vi "Notifer ControlThread.vi"() -> ()   [LabVIEW 2015]
panel:
  out "Waveform Chart 2":dbl(graph)
  out "Waveform Chart":dbl(graph)
  in  "stop":bool
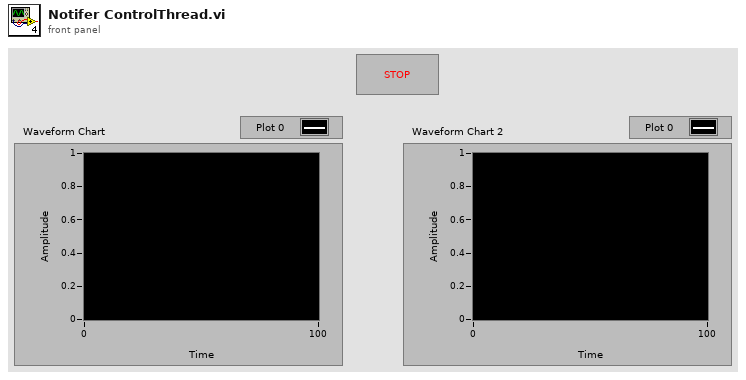
[diagram p1: front panel]
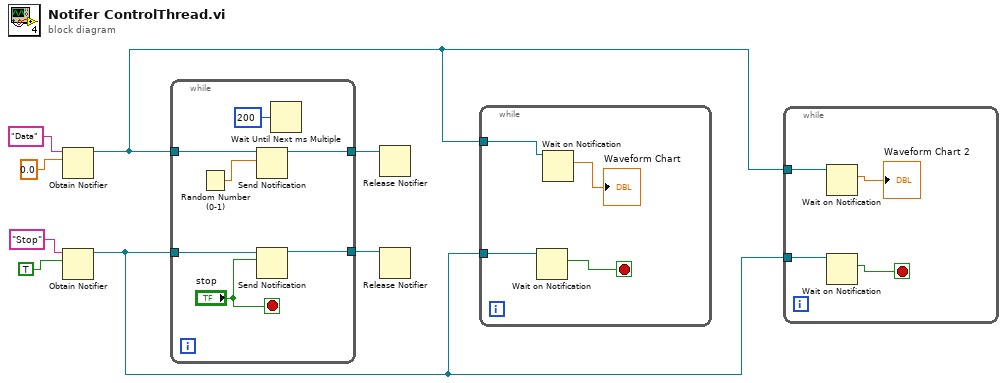
[diagram p0: block diagram]
diagram:
  n1 = Obtain Notifier(name (unnamed)="Data", notification data type=0.0 ("Waveform Chart")) -> (notifier out=w2:refnum<notifier>)  [unwired: 2 in, 2 out]
  n2 = Obtain Notifier(name (unnamed)="Stop", notification data type=TRUE) -> (notifier out=w1:refnum<notifier>)  [unwired: 2 in, 2 out]
  n3 = while {
    tunnel: w2 -> [w15]
    tunnel: w1 -> [w13]
    tunnel: [w14] -> w4
    tunnel: [w12] -> w3
    stop <- "stop" stop-if-true
    n4 = Random Number (0-1)() -> (number: 0 to 1=w11:dbl)
    n5 = Send Notification(notification=w11, notifier=w15) -> (notifier out=w14:refnum<notifier>)  [unwired: 1 in, 1 out]
    n6 = Send Notification(notification="stop", notifier=w13) -> (notifier out=w12:refnum<notifier>)  [unwired: 1 in, 1 out]
    n7 = Wait Until Next ms Multiple(millisecond multiple=u32 200) -> ()  [unwired: 1 out]
  }
  n8 = Release Notifier(notifier=w4) -> ()  [unwired: 2 in, 3 out]
  n9 = Release Notifier(notifier=w3) -> ()  [unwired: 2 in, 3 out]
  n10 = while {
    tunnel: w2 -> [w19]
    tunnel: w1 -> [w17]
    stop <- w16 stop-if-true
    n11 = Wait on Notification(notifier=w17) -> (notification=w16:bool)  [unwired: 3 in, 3 out]
    n12 = Wait on Notification(notifier=w19) -> (notification=→"Waveform Chart":dbl)  [unwired: 3 in, 3 out]
  }
  n13 = while {
    tunnel: w2 -> [w23]
    tunnel: w1 -> [w21]
    stop <- w20 stop-if-true
    n14 = Wait on Notification(notifier=w23) -> (notification=→"Waveform Chart 2":dbl)  [unwired: 3 in, 3 out]
    n15 = Wait on Notification(notifier=w21) -> (notification=w20:bool)  [unwired: 3 in, 3 out]
  }
